vi "Read Event.vi"(8 "error in (no error)":errorcluster caption="entrée d'erreur (pas d'erreur)", 11 "Class Event Shielding Box en entrée":refnum<class "Class Event Shielding Box.lvclass">) -> (0 "error out":errorcluster caption="sortie d'erreur", 3 "Class Event Shielding Box en sortie":refnum<class "Class Event Shielding Box.lvclass">)   [LabVIEW 2020, in "Library Instrument & Equipement.lvlib" / "Library Event.lvlib" / "Class Event Shielding Box.lvclass"]
uses:
  Class Event Shielding Box.lvclass
  C:/Users/ngarcin/OneDrive - Altyor/Standard TB/Class/Core/Actors/Actor_EventStart/Classe Event (Default)/Class Event (Default).lvclass
  JSON API/JSON Value/Set from JSON string.vi
  Instrument/Instrument (Default)/Class Instrument (Default).lvclass
  JSON API/JSON Value/JSON Value.lvclass
  Class Event Shielding Box.lvclass/Class Event Shielding Box.ctl
  JSON API/Variant JSON/Variant JSON.lvlib
  JSON API/Get Polymorphic/JSON GetSet.lvlib
panel:
  in  "Status":enum16{"Erreur", "Close", "Open"}(ring)
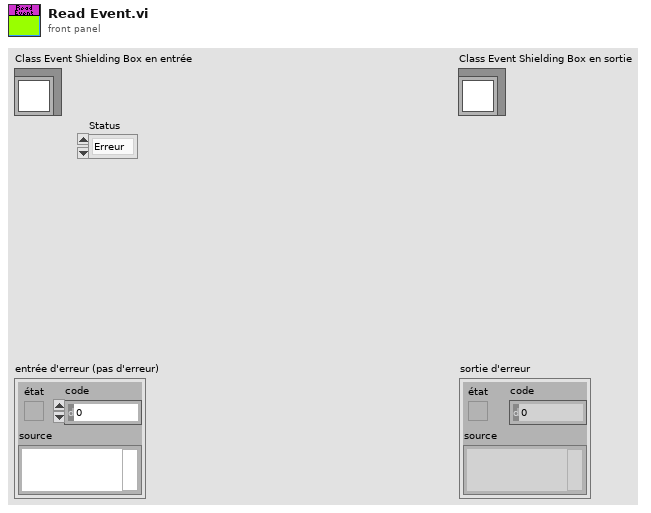
[diagram p1: front panel]
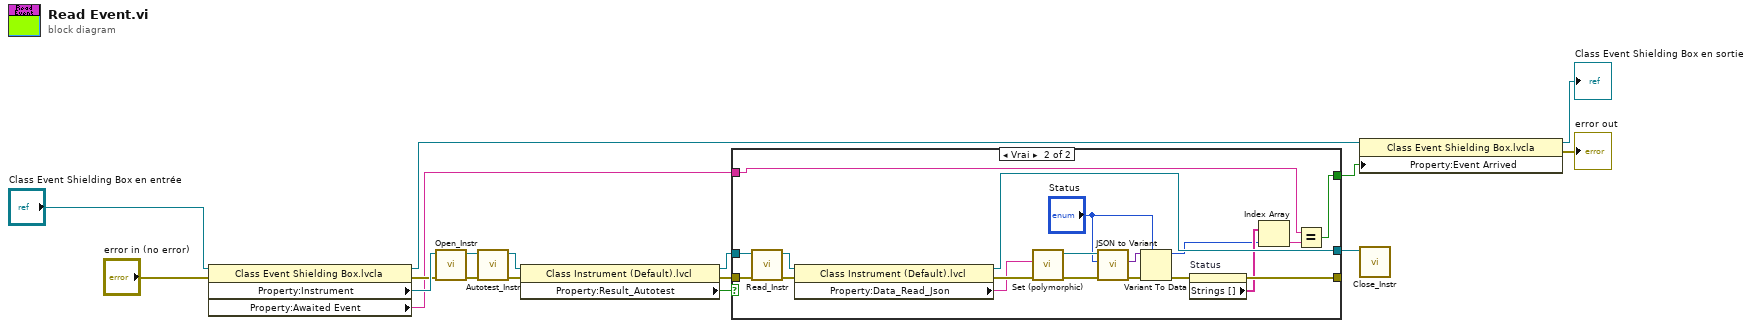
[diagram p0: block diagram]
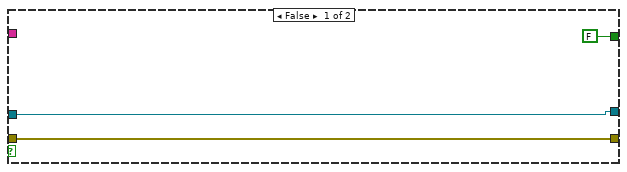
[diagram p2: hidden frame]
diagram:
  n1 = property class="Class Event Shielding Box.lvcla"(reference="Class Event Shielding Box en entrée", error in="error in (no error)") -> (reference out=w5:refnum<class "Class Event Shielding Box.lvclass">, error out=w9:errorcluster, "Property:Instrument"=w15:refnum<class "Class Instrument (Default).lvclass">, "Property:Awaited Event"=w1:string)
  n2 = call-dynamic "Open_Instr.vi"("error in (no error)"=w9, "Class Multimeter (Default) en entrée"=w15) -> ("error out"=w10:errorcluster, "Class Multimeter (Default) en sortie"=w14:refnum<class "Class Instrument (Default).lvclass">)  [unwired: 8 in]
  n3 = call-dynamic "Autotest_Instr.vi"("error in (no error)"=w10, "Class Instrument (Default) en entrée"=w14) -> ("error out"=w11:errorcluster, "Class Instrument (Default) en sortie"=w13:refnum<class "Class Instrument (Default).lvclass">)  [unwired: 8 in]
  n4 = property class="Class Instrument (Default).lvcl"(reference=w13, error in=w11) -> (reference out=w7:refnum<class "Class Instrument (Default).lvclass">, error out=w8:errorcluster, "Property:Result_Autotest"=w12:bool)
  n5 = case shown="Vrai" w12 {
    tunnel: w8 -> [w19 w39]
    tunnel: w7 -> [w20 w38]
    tunnel: [w20 w35] -> w6
    tunnel: [w19 w26] -> _
    tunnel: [FALSE w21] -> w2
    tunnel: w1 -> [_ w22]
    frame False {
    }
    frame True {
      n6 = call-dynamic "Read_Instr.vi"("error in (no error)"=w39, "Class Instrument (Default) en entrée"=w38) -> ("error out"=w36:errorcluster, "Class Instrument (Default) en sortie"=w37:refnum<class "Class Instrument (Default).lvclass">)  [unwired: 8 in]
      n7 = property class="Class Instrument (Default).lvcl"(reference=w37, error in=w36) -> (reference out=w35:refnum<class "Class Instrument (Default).lvclass">, error out=w29:errorcluster, "Property:Data_Read_Json"=w28:string)
      n8 = call-poly "Set (polymorphic).vi"("error in (no error)"=w29, "JSON stream"=w28) -> ("error out"=w33:errorcluster, "JSON Value out"=w31:refnum<class "JSON Value.lvclass">)  [unwired: 7 in, 1 out]
      n9 = call "JSON to Variant.vi"("error in (no error)"=w33, "Variant (Data Type)"="Status", "JSON Value"=w31) -> ("error out"=w32:errorcluster, "Variant out"=w34:variant)  [unwired: 7 in]
      n10 = Variant To Data(error in=w32, type="Status", Variant=w34) -> (data=w24:enum16{"Erreur", "Close", "Open"}, error out=w27:errorcluster)
      n11 = property on="Status" class="Énum (strict)"(error in=w27) -> (error out=w26:errorcluster, "Strings []"=w25:string[])  [unwired: 1 in, 1 out]
      n12 = Index Array(array=w25, index=w24) -> (element=w23:string)
      n13 = Equal?(x=w22, y=w23) -> (x = y?=w21:bool)
    }
  }
  n14 = property class="Class Event Shielding Box.lvcla"(reference=w5, "Property:Event Arrived"=w2) -> (reference out=→"Class Event Shielding Box en sortie":refnum<class "Class Event Shielding Box.lvclass">, error out=→"error out":errorcluster)  [unwired: 1 in]
  n15 = call-dynamic "Close_Instr.vi"("Class Instrument (Default) en entrée"=w6) -> ()  [unwired: 9 in, 2 out]
